vi "AnalyzeBlobs.vi"(9 "Vision Target":enum16{"Pegs", "Gears"}(ring), 10 "Blob Data":T2, 11 "Image In":T3) -> (2 "Target Data":T1, 3 "Image Out":T3)   [LabVIEW 2016]
uses:
  <vilib>/vision/Image Controls.llb/IMAQ Image.ctl
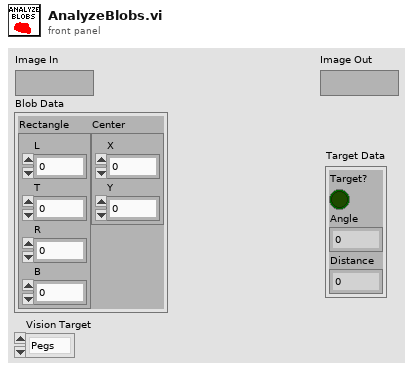
[diagram p1: front panel]
types:
  T1 = cluster{"Target?":bool, "Angle":dbl, "Distance":dbl}
  T2 = cluster{"Rectangle":cluster{"L":dbl, "T":dbl, "R":dbl, "B":dbl}, "Center":cluster{"X":dbl, "Y":dbl}}
  T3 = typedef "IMAQ Image.ctl" = refnum<image>
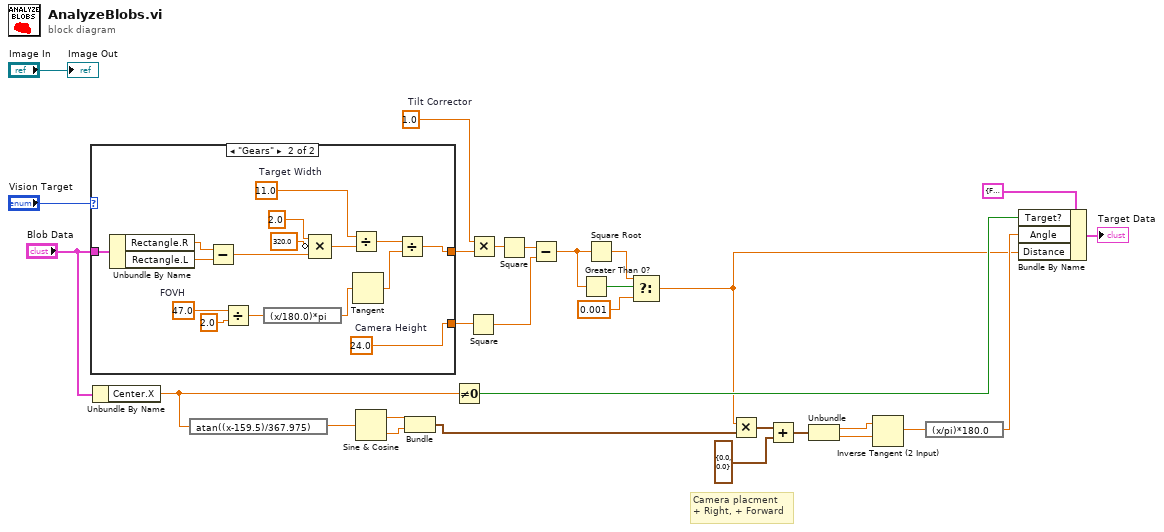
[diagram p0: block diagram]
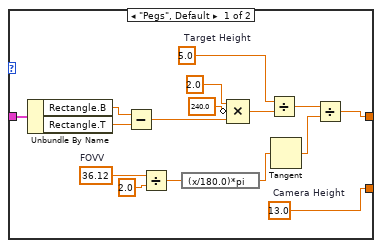
[diagram p2: hidden frame]
diagram:
  w27 = 1.0  # Tilt Corrector
  # "Camera placment\n+ Right, + Forward"
  n1 = case shown="\"Gears\"" "Vision Target" {
    tunnel: "Blob Data" -> [w45 w61]
    tunnel: [w35 w51] -> w26
    tunnel: [w34 w50] -> w24
    frame "Pegs", Default {
      w34 = 13.0  # Camera Height
      w40 = 36.12  # FOVV
      w31 = 5.0  # Target Height
      n2 = Unbundle By Name(w45) -> ("Rectangle.B"=w43:dbl, "Rectangle.T"=w44:dbl)
      n3 = Subtract(x=w43, y=w44) -> (x-y=w41:dbl)
      n4 = Divide(x=w40, y=2.0) -> (x/y=w38:dbl)
      n5 = expression code="(x/180.0)*pi" ("degrees to radians")(w38) -> (w37:dbl)
      n6 = Compound Arithmetic op=MULTIPLY(2.0 ("value"), invert 240.0 ("value"), w41) -> (w32:dbl)
      n7 = Divide(x=w31, y=w32) -> (x/y=w30:dbl)
      n8 = Tangent(1:w37) -> (0:w36:dbl)
      n9 = Divide(x=w30, y=w36) -> (x/y=w35:dbl)
    }
    frame "Gears" {
      w50 = 24.0  # Camera Height
      w56 = 47.0  # FOVH
      w47 = 11.0  # Target Width
      n10 = Unbundle By Name(w61) -> ("Rectangle.R"=w59:dbl, "Rectangle.L"=w60:dbl)
      n11 = Subtract(x=w59, y=w60) -> (x-y=w57:dbl)
      n12 = Divide(x=w56, y=2.0) -> (x/y=w54:dbl)
      n13 = expression code="(x/180.0)*pi" ("degrees to radians")(w54) -> (w53:dbl)
      n14 = Compound Arithmetic op=MULTIPLY(2.0 ("value"), invert 320.0 ("value"), w57) -> (w48:dbl)
      n15 = Divide(x=w47, y=w48) -> (x/y=w46:dbl)
      n16 = Tangent(1:w53) -> (0:w52:dbl)
      n17 = Divide(x=w46, y=w52) -> (x/y=w51:dbl)
    }
  }
  n18 = Unbundle By Name("Blob Data") -> ("Center.X"=w17:dbl)
  n19 = expression code="atan((x-159.5)/367.975)" ("degrees to radians")(w17) -> (w16:dbl)
  n20 = Sine & Cosine(0:w16) -> (1:w15:dbl, 2:w14:dbl)
  n21 = Bundle(w15, w14) -> (w13:cluster{dbl, dbl})  [unwired: 1 in]
  n22 = Not Equal To 0?(x=w17) -> (x != 0?=w18:bool)
  n23 = Square(x=w24) -> (x^2=w22:dbl)
  n24 = Multiply(x=w27, y=w26) -> (x*y=w25:dbl)
  n25 = Square(x=w25) -> (x^2=w23:dbl)
  n26 = Subtract(x=w23, y=w22) -> (x-y=w5:dbl)
  n27 = Greater Than 0?(x=w5) -> (x > 0?=w4:bool)
  n28 = Square Root(x=w5) -> (sqrt(x)=w2:dbl)
  n29 = Select(t=w2, s=w4, f=0.001) -> (s? t:f=w1:dbl)
  n30 = Multiply(x=w1, y=w13) -> (x*y=w12:cluster{dbl, dbl})
  n31 = Add(x=w12, y=cluster{dbl, dbl} {0.0, 0.0}) -> (x+y=w10:cluster{dbl, dbl})
  n32 = Unbundle(w10) -> (w9:dbl, w8:dbl)
  n33 = Inverse Tangent (2 Input)(1:w8, 2:w9) -> (0:w7:dbl)
  n34 = expression code="(x/pi)*180.0" ("radians to degrees")(w7) -> (w6:dbl)
  n35 = Bundle By Name(cluster=T1 {"Target?"=FALSE, "Angle"=0.0, "Distance"=0.0} ("Target Data"), "Target?"=w18, "Angle"=w6, "Distance"=w1) -> (→"Target Data":T1)
  "Image Out" <- "Image In"
